vi "u32 queue.vi"(8 "error in (no error)":errorcluster caption="エラー入力（エラーなし）", 10 "value in":u32, 11 "FGV Mode":T1=enum."Get") -> (0 "error out":errorcluster caption="エラー出力", 2 "value out":u32[](array[numeric]))   [LabVIEW 2018]
uses:
  FGV Mode.ctl
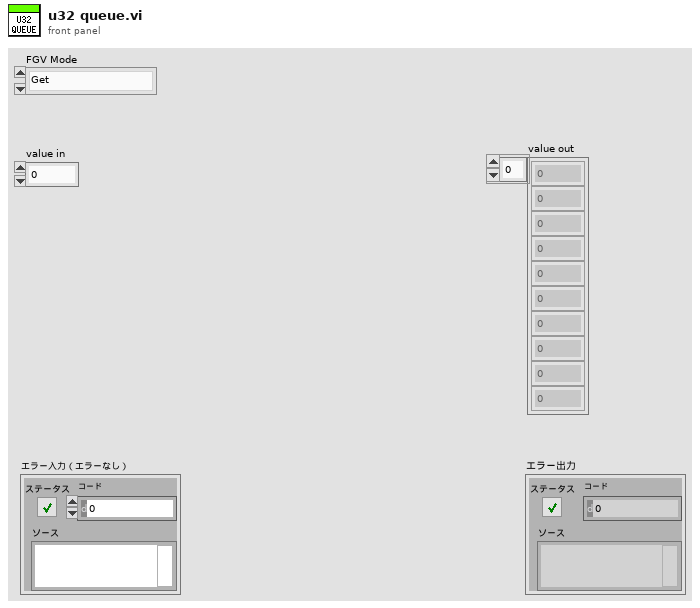
[diagram p1: front panel]
types:
  T1 = typedef "FGV Mode.ctl" = enum16{"None", "Init", "Set", "Get", "Update", "Clear"}
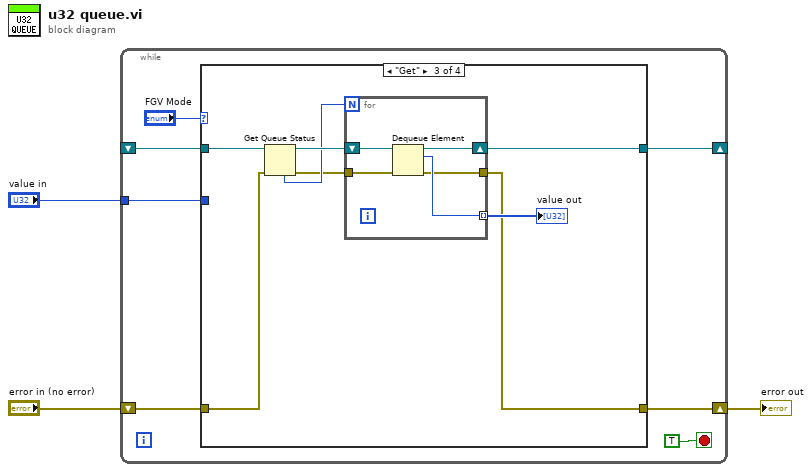
[diagram p0: block diagram]
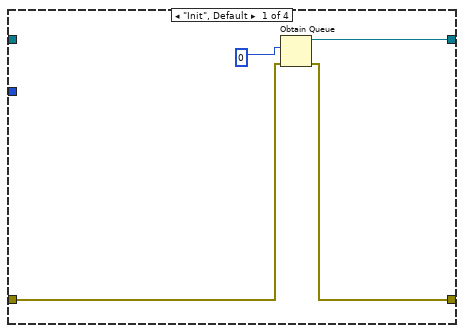
[diagram p2: hidden frame]
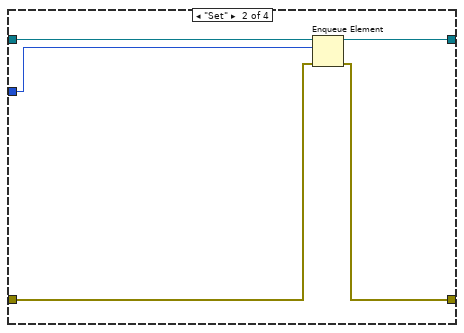
[diagram p3: hidden frame]
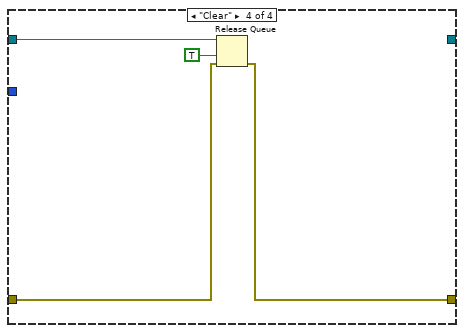
[diagram p4: hidden frame]
diagram:
  n1 = while {
    shift-right: [w8] -> w2
    shift-left: "error in (no error)" -> [w9]
    shift-right: [w6] -> _
    shift-left: _ -> [w5]
    tunnel: "value in" -> [w4]
    stop <- TRUE stop-if-true
    n2 = case shown="\"Get\"" "FGV Mode" {
      tunnel: w9 -> [w12 w16 w21 w34]
      tunnel: [w11 w15 w22 w33] -> w8
      tunnel: [w14 w18 w27 _] -> w6
      tunnel: w5 -> [_ w19 w26 w36]
      tunnel: w4 -> [_ w17 _ _]
      frame "Init", Default {
        n3 = Obtain Queue(element data type=u32 0 ("Elements Remaining"), error in (no error)=w12) -> (queue out=w14:refnum<queue>, error out=w11:errorcluster)  [unwired: 3 in, 1 out]
      }
      frame "Set" {
        n4 = Enqueue Element(queue=w19, element=w17, error in (no error)=w16) -> (queue out=w18:refnum<queue>, error out=w15:errorcluster)  [unwired: 1 in, 1 out]
      }
      frame "Get" {
        n5 = Get Queue Status(queue=w26, error in (no error)=w21) -> (queue out=w25:refnum<queue>, error out=w20:errorcluster, # elements in queue=w24:i32)  [unwired: 1 in, 5 out]
        n6 = for {
          N: w24 -> [_]
          shift-right: [w32] -> w27
          shift-left: w25 -> [w31]
          tunnel: [w30] -> w23 mode=indexing
          tunnel: w20 -> [w29]
          tunnel: [w28] -> w22
          n7 = Dequeue Element(queue=w31, error in (no error)=w29) -> (queue out=w32:refnum<queue>, element=w30:u32, error out=w28:errorcluster)  [unwired: 1 in, 1 out]
        }
        "value out" <- w23
      }
      frame "Clear" {
        n8 = Release Queue(queue=w36, force destroy? (F)=TRUE ("破棄を強制? (F)"), error in (no error)=w34) -> (error out=w33:errorcluster)  [unwired: 2 out]
      }
    }
  }
  "error out" <- w2
